vi "Variant to Class.vi"(8 "error in (no error)":errorcluster, 10 "Data in":variant, 11 "CI Project in":refnum<class "CI Project.lvclass">) -> (0 "error out":errorcluster, 2 "Data Out":variant, 3 "CI Project out":refnum<class "CI Project.lvclass">)   [LabVIEW 2014, in "CI Project.lvclass"]
uses:
  CI Project.lvclass
  CI Project.lvclass/CI Project.ctl
  Build Job/Build Job.lvclass
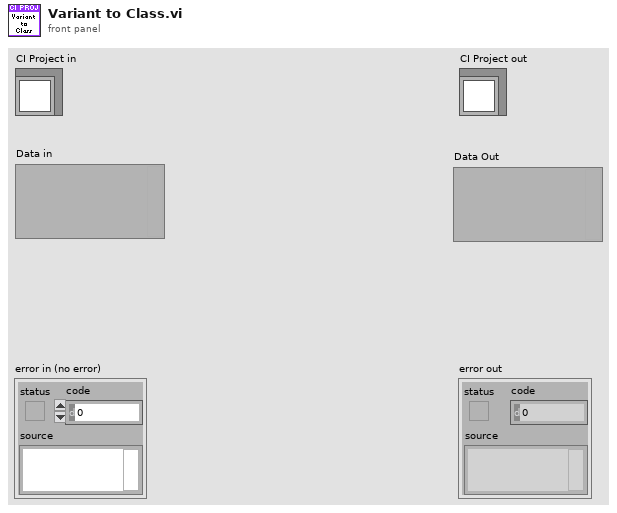
[diagram p1: front panel]
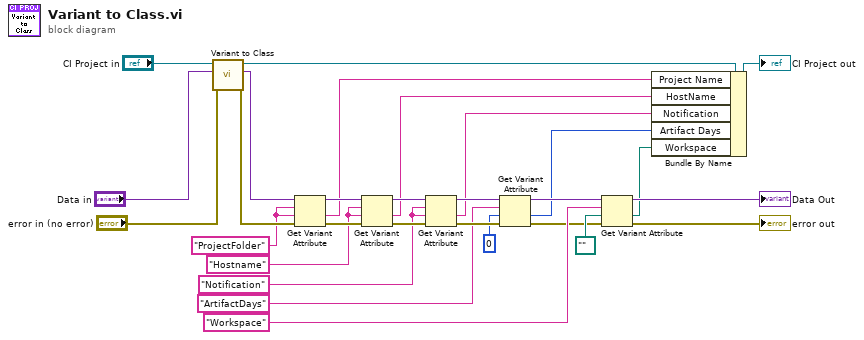
[diagram p0: block diagram]
diagram:
  w13 = "Hostname"
  w14 = "Notification"
  w15 = "ProjectFolder"
  n1 = call-parent "Variant to Class.vi"("error in (no error)"="error in (no error)", "Data in"="Data in", "Build Job in"="CI Project in") -> ("error out"=w25:errorcluster, "Data Out"=w22:variant, "Build Job out"=w29:refnum<class "CI Project.lvclass">)  [unwired: 6 in]
  n2 = Get Variant Attribute(Variant=w22, name=w15, default value (empty Variant)=w15, error in=w25) -> (duplicate Variant=w20:variant, value=w10:string, error out=w23:errorcluster)  [unwired: 1 out]
  n3 = Get Variant Attribute(Variant=w20, name=w13, default value (empty Variant)=w13, error in=w23) -> (duplicate Variant=w19:variant, value=w9:string, error out=w21:errorcluster)  [unwired: 1 out]
  n4 = Get Variant Attribute(Variant=w19, name=w14, default value (empty Variant)=w14, error in=w21) -> (duplicate Variant=w18:variant, value=w8:string, error out=w24:errorcluster)  [unwired: 1 out]
  n5 = Get Variant Attribute(Variant=w18, name="ArtifactDays", default value (empty Variant)=0 ("Artifact Days"), error in=w24) -> (duplicate Variant=w17:variant, value=w7:i32, error out=w2:errorcluster)  [unwired: 1 out]
  n6 = Get Variant Attribute(Variant=w17, name="Workspace", default value (empty Variant)=path "", error in=w2) -> (duplicate Variant=→"Data Out":variant, value=w3:path, error out=→"error out":errorcluster)  [unwired: 1 out]
  n7 = Bundle By Name(cluster=w29, "Project Name"=w10, "HostName"=w9, "Notification"=w8, "Artifact Days"=w7, "Workspace"=w3) -> (→"CI Project out":refnum<class "CI Project.lvclass">)
